vi "FormPopup.vi"(8 "エラー入力（エラーなし）":errorcluster, 11 "VI入力":refnum<vi>) -> (0 "エラー出力":errorcluster)   [LabVIEW 2014]
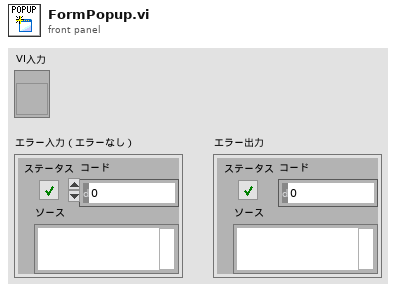
[diagram p1: front panel]
types:
  T1 = enum32{"Invalid", "Standard", "Closed", "Hidden", "Minimized", "Maximized"}
  T2 = enum32{"Bad", "Idle", "Run top level", "Running"}
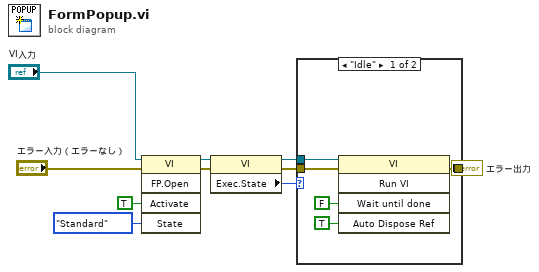
[diagram p0: block diagram]
diagram:
  n1 = invoke class="VI" method="FP.Open"(reference="VI入力", error in="エラー入力（エラーなし）", "Activate"=TRUE ("アクティブ化?"), "State"=T1."Standard" ("状態")) -> (reference out=w3:refnum<vi>, error out=w4:errorcluster)  [unwired: 1 in, 3 out]
  n2 = property class="VI"(reference=w3, error in=w4) -> (error out=w7:errorcluster, "Exec.State"=w5:T2)  [unwired: 1 out]
  n3 = case shown="\"Idle\"" w5 {
    tunnel: w3 -> [w12 _]
    tunnel: w7 -> [w11 w15]
    tunnel: [w10 w15] -> w8
    frame "Idle" {
      n4 = invoke class="VI" method="Run VI"(reference=w12, error in=w11, "Wait until done"=FALSE ("終了まで待機"), "Auto Dispose Ref"=TRUE ("リファレンスを自動破棄")) -> (error out=w10:errorcluster)  [unwired: 1 in, 4 out]
    }
    frame Default {
    }
  }
  "エラー出力" <- w8
